vi "New Table with Cell Styles.vi"(6 "Cell.Styles":refnum<class "Style.lvclass">[][](array[class]), 7 "xwpfTable Type":refnum<class "xwpfTable.lvclass">, 8 "error in (no error)":errorcluster, 10 "Table":string[][](array[string]), 11 "Table Ref":refnum<k24>) -> (0 "error out":errorcluster, 3 "xwpfTable out":refnum<class "xwpfTable.lvclass">)   [LabVIEW 2017, in "Word_Specific.lvlib" / "xwpfTable.lvclass"]
uses:
  xwpfTable.lvclass
  C:/Users/Neo/Desktop/Dev_Tools_BR/LabVIEW_NPOI/src/lib/NPOI 2.1.1/NPOI.OOXML.dll
  lib/NPOI 2.1.1/NPOI.OOXML.dll
  Styles/Style/Style.lvclass
  xwpfTable.lvclass/xwpfTable.ctl
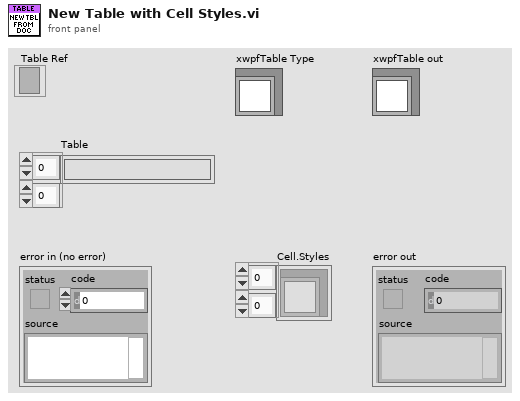
[diagram p1: front panel]
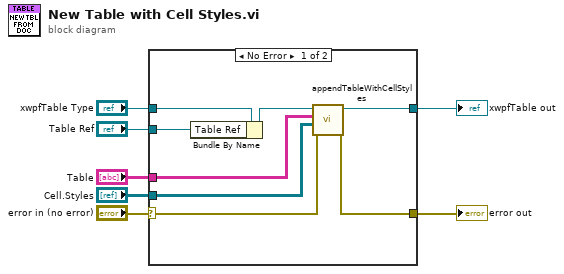
[diagram p0: block diagram]
diagram:
  n1 = case shown="No Error" "error in (no error)" {
    selector: "error in (no error)" -> [w10 w17]
    tunnel: [w9 w17] -> w6
    tunnel: [w12 w16] -> w4
    tunnel: "xwpfTable Type" -> [w15 w16]
    tunnel: "Table Ref" -> [w14 _]
    tunnel: "Table" -> [w11 _]
    tunnel: "Cell.Styles" -> [w8 _]
    frame No Error {
      n2 = Bundle By Name(cluster=w15, "Table Ref"=w14) -> (w13:refnum<class "xwpfTable.lvclass">)
      n3 = call "appendTableWithCellStyles.vi"("error in (no error)"=w10, "Cell.Styles"=w8, "Table"=w11, "xwpfTable in"=w13) -> ("error out"=w9:errorcluster, "xwpfTable out"=w12:refnum<class "xwpfTable.lvclass">)  [unwired: 6 in]
    }
    frame Error {
    }
  }
  "error out" <- w6
  "xwpfTable out" <- w4
